vi "Escáner.vi"(9 "Fabricante":u16(ring) items=["PowerFlex", "Schneider", "Delta", "ABB", "LS Electric"], 10 "Puerto COM":refnum<visa-resource-name>) -> (0 "error out":errorcluster, 1 "Datos":i32[](array[numeric]), 2 "VFD encontrado":bool, 3 "Modbus master out":refnum<class "Modbus Master.lvclass">, 5 "Timeout":i32 format="%.0f mseg.")   [LabVIEW 2013]
uses:
  <vilib>/NI/Modbus Library/API/Master/Modbus Master.lvclass
  Variables globales/Temporales.vi
  <vilib>/NI/Modbus Library/API/Wrapper/Create Serial Master.vi
  <vilib>/NI/Modbus Library/API/Wrapper/API Main.lvlib
panel:
  out "Avance":i32
  out "Mensaje":string
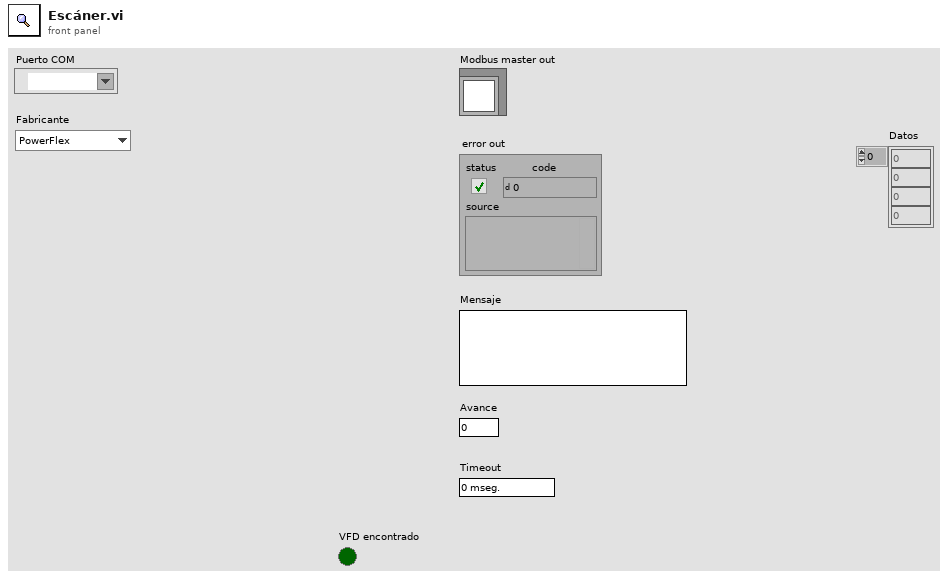
[diagram p1: front panel]
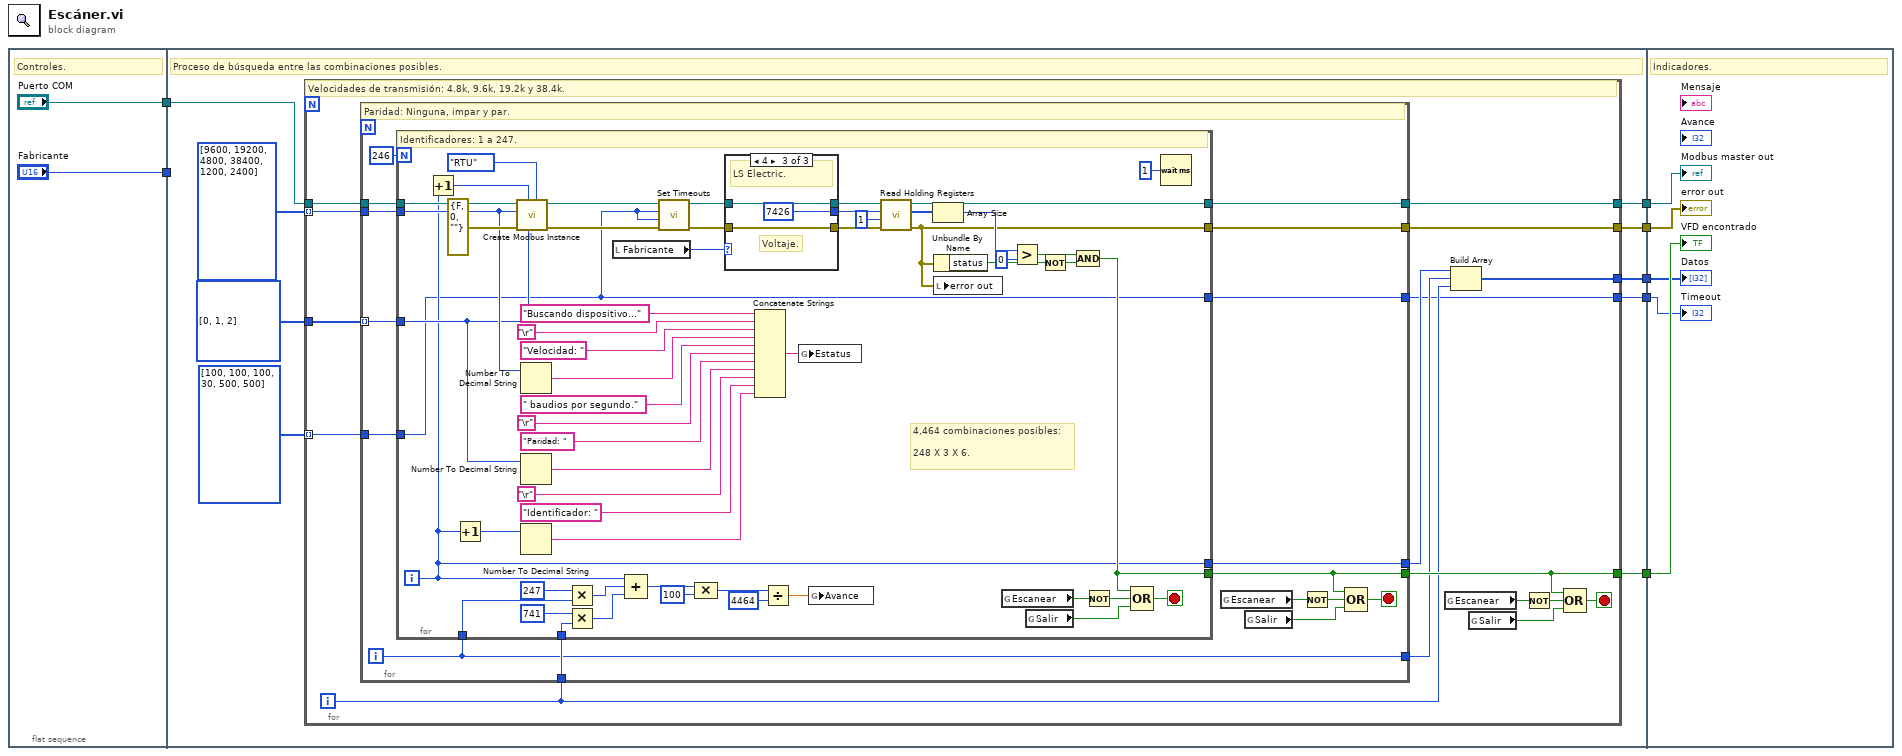
[diagram p0: block diagram]
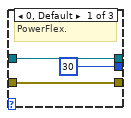
[diagram p2: hidden frame]
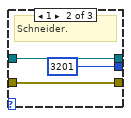
[diagram p3: hidden frame]
diagram:
  n1 = flat-sequence {
    tunnel: ["Puerto COM"] -> w7
    tunnel: ["Fabricante"] -> w2
    tunnel: w7 -> [w16]
    tunnel: [w15] -> w6
    tunnel: [w14] -> w5
    tunnel: [w13] -> w4
    tunnel: [w12] -> w3
    tunnel: w2 -> [_]
    tunnel: [w10] -> w1
    tunnel: w6 -> [w119]
    tunnel: w5 -> [w118]
    tunnel: w4 -> [w117]
    tunnel: w3 -> [w116]
    tunnel: w1 -> [w115]
    frame #0 {
      # "Controles."
    }
    frame #1 {
      w17 = u16[] [0, 1, 2] items=["None", "Odd", "Even", "Mark", "Space"]
      # "Proceso de búsqueda entre las combinaciones posibles."
      n2 = for {
        tunnel: i32[] [9600, 19200, 4800, 38400, 1200, 2400] -> [w33] mode=indexing
        tunnel: w17 -> [w34]
        tunnel: w16 -> [w32]
        tunnel: [w31] -> w15
        tunnel: [w30] -> w14
        tunnel: [w28] -> w13
        tunnel: [w24] -> w12
        tunnel: i32[] [100, 100, 100, 30, 500, 500] -> [w23] mode=indexing
        tunnel: [w22] -> w10
        i -> [w25]
        stop <- w29 stop-if-true
        # "Velocidades de transmisión: 4.8k, 9.6k, 19.2k y 38.4k."
        n3 = for {
          tunnel: w34 -> [w48] mode=indexing
          tunnel: w33 -> [w49]
          tunnel: w32 -> [w47]
          tunnel: [w46] -> w31
          tunnel: [w45] -> w30
          tunnel: [w43] -> w28
          tunnel: w25 -> [w42]
          tunnel: [w40] -> w26
          tunnel: [w41] -> w27
          tunnel: w23 -> [w39]
          tunnel: [w38] -> w22
          i -> [w40]
          stop <- w44 stop-if-true
          # "Paridad: Ninguna, impar y par."
          n4 = for {
            N: 246 -> [_]
            tunnel: w49 -> [w76]
            tunnel: w48 -> [w75]
            tunnel: w47 -> [w104]
            tunnel: [w97] -> w46
            tunnel: [w74] -> w45
            tunnel: [w90] -> w43
            tunnel: w40 -> [w69]
            tunnel: w42 -> [w66]
            tunnel: [w60] -> w41
            tunnel: w39 -> [w54]
            tunnel: [w54] -> w38
            i -> [w60]
            stop <- w91 stop-if-true
            # "4,464 combinaciones posibles:\n\n248 X 3 X 6."
            # "Identificadores: 1 a 247."
            n5 = Increment(x=w60) -> (x+1=w102:i32)
            n6 = Increment(x=w60) -> (x+1=w77:i32)
            n7 = call-poly <vilib>:"Create Modbus Instance.vi"("serial type"=enum16{"RTU", "ASCII"}."RTU", "parity (even)"=w75, "unit ID"=w102, "error in"=errorcluster {"status"=FALSE, "code"=0, "source"=""}, "baud rate"=w76, "VISA resource name"=w104) -> ("error out"=w99:errorcluster, "serial master instance"=w100:refnum<class "Modbus Master.lvclass">)  [unwired: 4 in]
            n8 = Number To Decimal String(number=w76) -> (decimal integer string=w81:string)  [unwired: 1 in]
            n9 = Number To Decimal String(number=w75) -> (decimal integer string=w80:string)  [unwired: 1 in]
            n10 = Number To Decimal String(number=w77) -> (decimal integer string=w79:string)  [unwired: 1 in]
            n11 = Multiply(x=247, y=w69) -> (x*y=w71:i32)
            n12 = Multiply(x=741, y=w66) -> (x*y=w67:i32)
            n13 = local read "Fabricante"() -> (w55:u16)
            n14 = Compound Arithmetic op=ADD(w60, w71, w67) -> (w65:i32)
            n15 = call <vilib>:"Set Timeouts.vi"("error in"=w99, "write operation timeout"=w54, "read operation timeout"=w54, "Modbus master in"=w100) -> ("error out"=w58:errorcluster, "Modbus master out"=w59:refnum<class "Modbus Master.lvclass">)  [unwired: 6 in]
            n16 = Compound Arithmetic op=MULTIPLY(w65, 100) -> (w63:i32)
            n17 = case shown="4" w55 {
              tunnel: w59 -> [w108 w111 w114]
              tunnel: w58 -> [w107 w110 w113]
              tunnel: [w108 w111 w114] -> w57
              tunnel: [w107 w110 w113] -> w105
              tunnel: [u16 30 ("starting address") u16 3201 ("starting address") u16 7426 ("starting address")] -> w56
              frame 0, Default {
                # "PowerFlex."
              }
              frame 1 {
                # "Schneider."
              }
              frame 4 {
                # "Voltaje."
                # "LS Electric."
              }
            }
            n18 = Concatenate Strings("Buscando dispositivo...", "\r", "Velocidad: ", w81, " baudios por segundo.", "\r", "Paridad: ", w80, "\r", "Identificador: ", w79) -> (w72:string)
            n19 = Divide(x=w63, y=4464) -> (x/y=w61:dbl)
            n20 = global write "Temporales.vi" "Estatus"(w72) -> ()
            n21 = global write "Temporales.vi" "Avance"(w61) -> ()
            n22 = call-dynamic "Read Holding Registers.vi"("error in"=w105, "number of inputs"=u16 1, "starting address"=w56, "Modbus master in"=w57) -> ("error out"=w74:errorcluster, "register values"=w94:u16[], "Modbus master out"=w97:refnum<class "Modbus Master.lvclass">)  [unwired: 5 in]
            n23 = Array Size(array=w94) -> (size(s)=w93:i32)
            n24 = Unbundle By Name(w74) -> ("status"=w92:bool)
            n25 = local write "error out"(w74) -> ()
            n26 = global read "Temporales.vi" "Escanear"() -> (w53:bool)
            n27 = Greater?(x=w93, y=0) -> (0:w95:bool)
            n28 = global read "Temporales.vi" "Salir"() -> (w51:bool)
            n29 = Not(x=w92) -> (.not. x?=w73:bool)
            n30 = Compound Arithmetic op=AND(w95, w73) -> (w90:bool)
            n31 = Not(x=w53) -> (.not. x?=w52:bool)
            n32 = Compound Arithmetic op=OR(w90, w52, w51) -> (w91:bool)
            n33 = Wait (ms)(milliseconds to wait=u32 1) -> ()  [unwired: 1 out]
          }
          n34 = global read "Temporales.vi" "Escanear"() -> (w36:bool)
          n35 = global read "Temporales.vi" "Salir"() -> (w35:bool)
          n36 = Not(x=w36) -> (.not. x?=w37:bool)
          n37 = Compound Arithmetic op=OR(w43, w37, w35) -> (w44:bool)
        }
        n38 = global read "Temporales.vi" "Escanear"() -> (w21:bool)
        n39 = Build Array(w27, w26, w25) -> (w24:i32[])
        n40 = global read "Temporales.vi" "Salir"() -> (w19:bool)
        n41 = Not(x=w21) -> (.not. x?=w20:bool)
        n42 = Compound Arithmetic op=OR(w28, w20, w19) -> (w29:bool)
      }
    }
    frame #2 {
      # "Indicadores."
      "error out" <- w118
      "Modbus master out" <- w119
      "VFD encontrado" <- w117
      "Datos" <- w116
      "Timeout" <- w115
    }
  }
